vi "fibonacci.vi"() -> ()   [LabVIEW 2017]
doc: "Generate nth number in the fibonacci series"
panel:
  in  "stop":bool
  out "Fn":i32
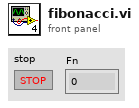
[diagram p1: front panel]
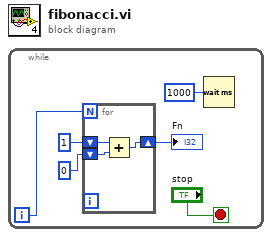
[diagram p0: block diagram]
diagram:
  n1 = while {
    i -> [w2]
    stop <- "stop" stop-if-true
    n2 = for {
      N: w2 -> [_]
      shift-right: [w8] -> w4
      shift-left: 1 -> [w9]
      shift-left: 0 -> [w7]
      n3 = Add(x=w9, y=w7) -> (x+y=w8:i32)
    }
    "Fn" <- w4
    n4 = Wait (ms)(milliseconds to wait=u32 1000) -> ()  [unwired: 1 out]
  }
